vi "FuncImg-Export full data-Core.vi"(8 "FOR loop index":i32, 9 "System Cluster":T4 {"ROI number" min=1 format="ROI %.0f"}, 10 "Input cluster":T3={"Channel A?"=FALSE, "MovCor enabled"=FALSE, "Cycle time-stamps (us)"=[], "Cycle length (us)"=0.0, "[Pixels in ROI]"=[], "Z-Stack Header data"={"Number of POI"=0, "Number of Miniscans"=0, "Number of Trials"=0, "Number of Cycles "=0, "# Averaged Frames"=0, "Laser power (%)"=0, "Pockels"=0.0, "Acquisition Length (sec)"=0.0, "Fill time (us)"=0.0, "DwellTime (us)"=0.0, "Miniscan Dwell time per pixel (us)"=0.0, "PMT 1"=0.0, "PMT 2"=0.0, "Back Apperture"=0.0, "Zoom"=0.0, "Number of Pixels in Miniscan"=0, "Frame Size"=200, "Field of View"=0.0, "X centre"=0.0, "Y centre"=0.0, "AOL Z"=0.0}, "[ROI Time (us)]"=[], "Path out"=path "", "Version index"=0} {"Z-Stack Header data"."Frame Size" items=["100X100"=100, "128X128"=128, "200X200"=200, "256X256"=256, "512X512"=512, "1024x1024"=1024, "2048x2048"=2048]; "Z-Stack Header data"."Back Apperture" format="%#.6g"; "Z-Stack Header data"."Pockels" format="%#.6g"; "Z-Stack Header data"."PMT 2" format="%#.6g"; "Z-Stack Header data"."PMT 1" format="%#.6g"; "Z-Stack Header data"."Miniscan Dwell time per pixel (us)" format="%#.6g"; "Z-Stack Header data"."Zoom" format="%#.6g"; "Z-Stack Header data"."DwellTime (us)" format="%#.6g"; "Z-Stack Header data"."Acquisition Length (sec)" format="%#.6g"; "Z-Stack Header data"."Fill time (us)" format="%#.6g"}, 11 "Exported tdms file":refnum<k34>) -> (0 "error out":errorcluster, 3 "Exported tdms file":refnum<k34>)   [LabVIEW 2017]
uses:
  xcontrol/Interface VIs/Interface typedefs/Interface-ROI selection cluster.ctl
  Typedefs/ROI ID Enum.ctl
  Experiment header interface/Typedefs/Header parameters cluster-Zstack.ctl
  Typedefs/Frame Size.ctl
panel:
  # "<--- Timeline data already decimated\n          for memory efficiency."
  # "Zstack header parameters"
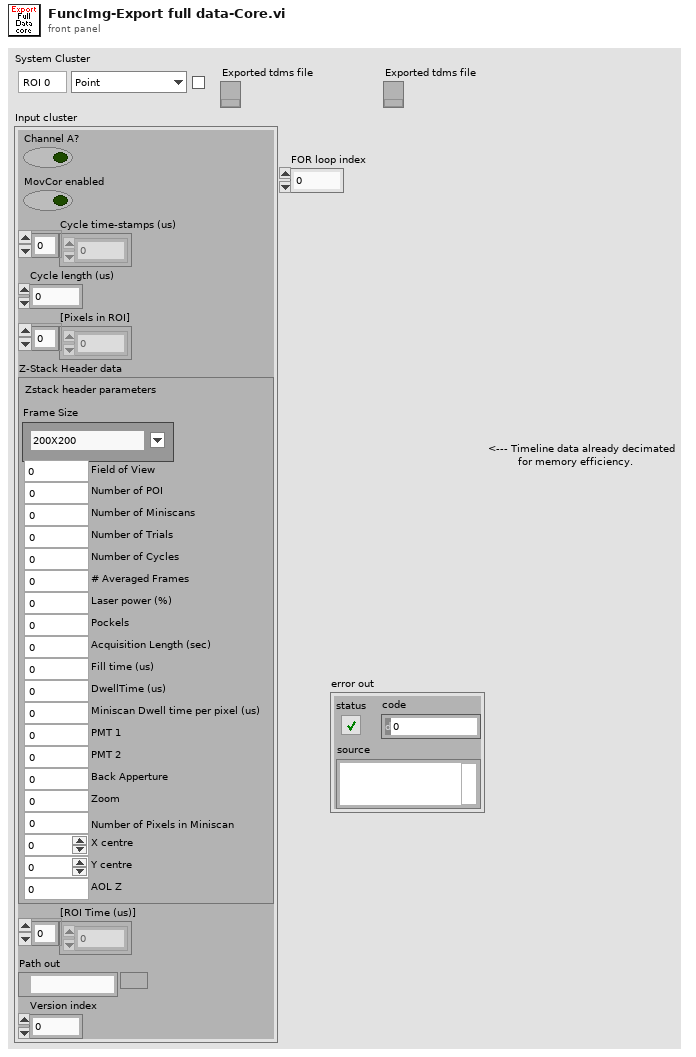
[diagram p1: front panel]
types:
  T1 = typedef "Header parameters cluster-Zstack.ctl" = cluster{"Number of POI":u16, "Number of Miniscans":u16, "Number of Trials":u16, "Number of Cycles ":u16, "# Averaged Frames":u16, "Laser power (%)":u8, "Pockels":dbl, "Acquisition Length (sec)":dbl, "Fill time (us)":dbl, "DwellTime (us)":dbl, "Miniscan Dwell time per pixel (us)":dbl, "PMT 1":dbl, "PMT 2":dbl, "Back Apperture":dbl, "Zoom":dbl, "Number of Pixels in Miniscan":u16, "Frame Size":T2, "Field of View":dbl, "X centre":dbl, "Y centre":dbl, "AOL Z":dbl}
  T2 = typedef "Frame Size.ctl" = u16
  T3 = cluster{"Channel A?":bool, "MovCor enabled":bool, "Cycle time-stamps (us)":dbl[], "Cycle length (us)":dbl, "[Pixels in ROI]":i32[], "Z-Stack Header data":T1, "[ROI Time (us)]":dbl[], "Path out":path, "Version index":i32}
  T4 = typedef "Interface-ROI selection cluster.ctl" = cluster{"ROI number":i32, "ROI ID":T5, "Visibility":bool}
  T5 = typedef "ROI ID Enum.ctl" = enum16{"Point", "MiniScan", "Comp. MiniScan", "Rectangle", "Comp. volume", "Arb. plane point"}
  T6 = typedef "Interface-ROI type enum.ctl" = enum16{"POI", "Mini-scan"}
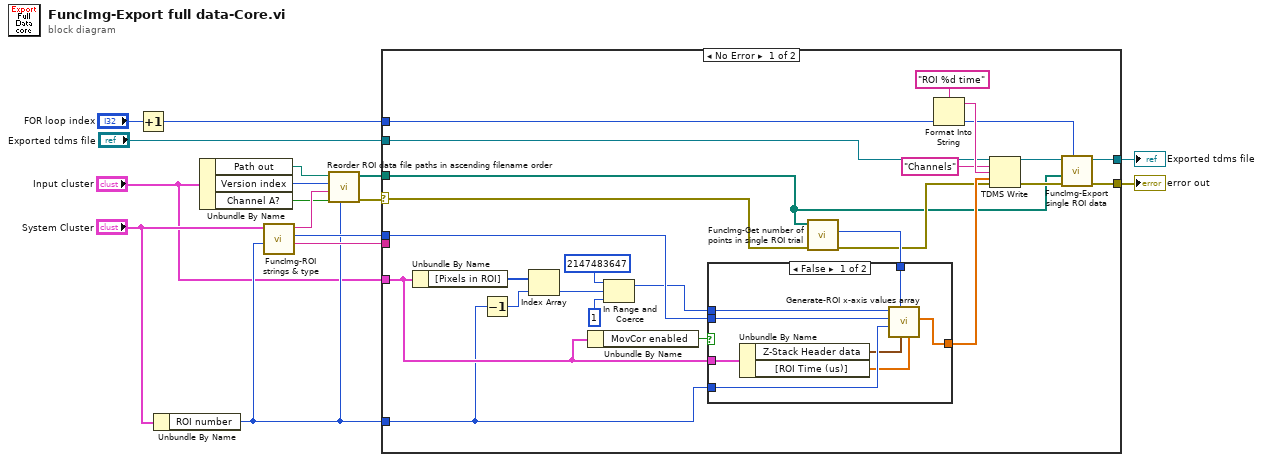
[diagram p0: block diagram]
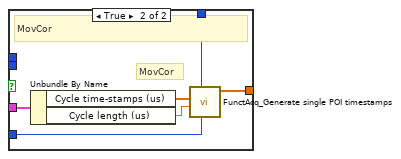
[diagram p2: hidden frame]
diagram:
  n1 = Increment(x="FOR loop index") -> (x+1=w1:i32)
  n2 = Unbundle By Name("System Cluster") -> ("ROI number"=w9:i32)
  n3 = Unbundle By Name("Input cluster") -> ("Path out"=w15:path, "Version index"=w16:i32, "Channel A?"=w12:bool)
  n4 = call "FuncImg-ROI strings & type.vi"("ROI number"=w9, "ROI visibility cluster"="System Cluster") -> ("Plot name"=w11:string, "ROI type"=w14:T6, "ROI ID string"=w13:string)  [unwired: 7 in]
  n5 = call "Reorder ROI data file paths in ascending filename order.vi"("ROI number"=w9, "Channel A?"=w12, "ROI ID string"=w13, "ROI file format version"=w16, "Dataset directory path"=w15) -> ("Error out"=w7:errorcluster, "Reordered file paths in ascending file-name order"=w5:path[])  [unwired: 5 in]
  n6 = case shown="No Error" w7 {
    selector: w7 -> [w29 w56]
    tunnel: w14 -> [w38 _]
    tunnel: w5 -> [w17 _]
    tunnel: w11 -> [_ _]
    tunnel: w9 -> [w31 _]
    tunnel: "Input cluster" -> [w32 _]
    tunnel: [w19 w56] -> w6
    tunnel: "Exported tdms file" -> [w24 w55]
    tunnel: w1 -> [w18 _]
    tunnel: [w21 w55] -> w2
    frame No Error {
      n7 = Unbundle By Name(w32) -> ("[Pixels in ROI]"=w39:i32[])
      n8 = Decrement(x=w31) -> (x-1=w37:i32)
      n9 = Index Array(array=w39, index=w37) -> (element=w33:i32)
      n10 = Unbundle By Name(w32) -> ("MovCor enabled"=w40:bool)
      n11 = In Range and Coerce(upper limit=2147483647, x=w33, lower limit=1) -> (coerced(x)=w36:i32)  [unwired: 1 out]
      n12 = call "FuncImg-Get number of points in single ROI trial.vi"("Error in"=w29, "Single ROI data files reorderedin ascending file-name order"=w17) -> ("Error out"=w23:errorcluster, "Number of data points in single POI (all trials)"=w30:i32)  [unwired: 8 in]
      n13 = case shown="False" w40 {
        tunnel: w38 -> [w48 _]
        tunnel: w36 -> [w47 _]
        tunnel: w31 -> [w46 w53]
        tunnel: w30 -> [w45 w54]
        tunnel: [w44 w52] -> w26
        tunnel: w32 -> [w43 w49]
        frame False {
          n14 = Unbundle By Name(w43) -> ("Z-Stack Header data"=w42:T1, "[ROI Time (us)]"=w41:dbl[])
          n15 = call "Generate-ROI x-axis values array.vi"("[ROI Time(us)]"=w41, "Header data"=w42, "Number of points in Y-axis array"=w45, "ROI number"=w46, "Type"=w48, "Pixels in ROI"=w47) -> ("ROI X-axis values array (sec)"=w44:sgl[])  [unwired: 5 in]
        }
        frame True {
          # "MovCor"
          # "MovCor"
          n16 = Unbundle By Name(w49) -> ("Cycle time-stamps (us)"=w51:dbl[], "Cycle length (us)"=w50:dbl)
          n17 = call "FunctAcq_Generate single POI timestamps.vi"("ROI number"=w53, "Number of data points in single POI (all trials)"=w54, "Funct Acq cycle length (us)"=w50, "Single funct.acq cycle time-stamps (us)"=w51) -> ("Full timestamps array for single POI (sec)"=w52:sgl[])  [unwired: 7 in]
        }
      }
      n18 = Format Into String(format string="ROI %d time", w18) -> (resulting string=w27:string)  [unwired: 2 in, 1 out]
      n19 = TDMS Write(0:w24, 5:"Channels" ("group name"), 7:w27, 9:w26, 11:w23) -> (4:w22:refnum<k34>, 15:w20:errorcluster)  [unwired: 1 in, 2 out]
      n20 = call "FuncImg-Export single ROI data.vi"("ROI number"=w18, "Error in"=w20, "Single ROI data files reorderedin ascending file-name order"=w17, "Exported tdms file"=w22) -> ("Error out"=w19:errorcluster, "Exported tdms file"=w21:refnum<k34>)  [unwired: 5 in, 1 out]
    }
    frame Error {
    }
  }
  "error out" <- w6
  "Exported tdms file" <- w2
